vi "36DUT Plot From Spread Sheet Ver1.5a.vi"(6 "Plot":T1(ring), 7 "No of Rows":i32=10496, 8 "error in (no error)":errorcluster, 10 "Bank":i32(ring) items=["C1", "C2", "C3", "D_C1", "D_C2", "D_C3", "D_B1_C1", "D_B1_C2", "D_B1_C3"], 11 "file path (dialog if empty)":path) -> (0 "error out":errorcluster, 3 "Delta C_Min Plot":dbl[][](graph) caption="(Y) Multi Plot 2")   [LabVIEW 2012]
uses:
  <vilib>/Utility/file.llb/Read From Spreadsheet File (string).vi
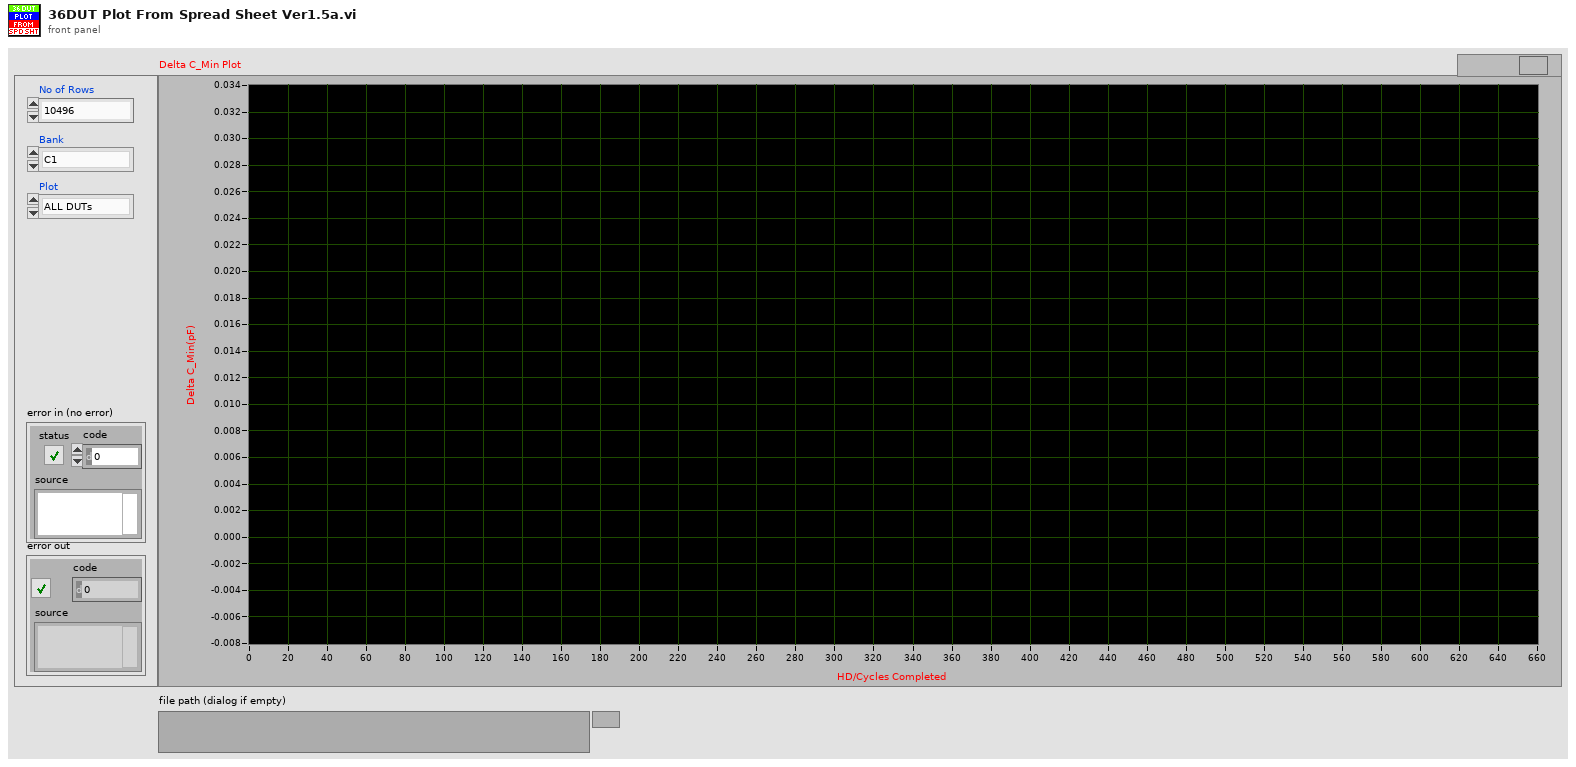
[diagram p1: front panel]
types:
  T1 = enum16{"ALL DUTs", "DUT 01", "DUT 02", "DUT 03", "DUT 04", "DUT 05", "DUT 06", "DUT 07", "DUT 08", "DUT 09", "DUT 10", "DUT 11", "DUT 12", "DUT 13", "DUT 14", "DUT 15", "DUT 16", "DUT 17", "DUT 18", "DUT 19", "DUT 20", "DUT 21", "DUT 22", "DUT 23", "DUT 24", "DUT 25", "DUT 26", "DUT 27", "DUT 28", "DUT 29", "DUT 30", "DUT 31", "DUT 32", "DUT 33", "DUT 34", "DUT 35", "DUT 36"}
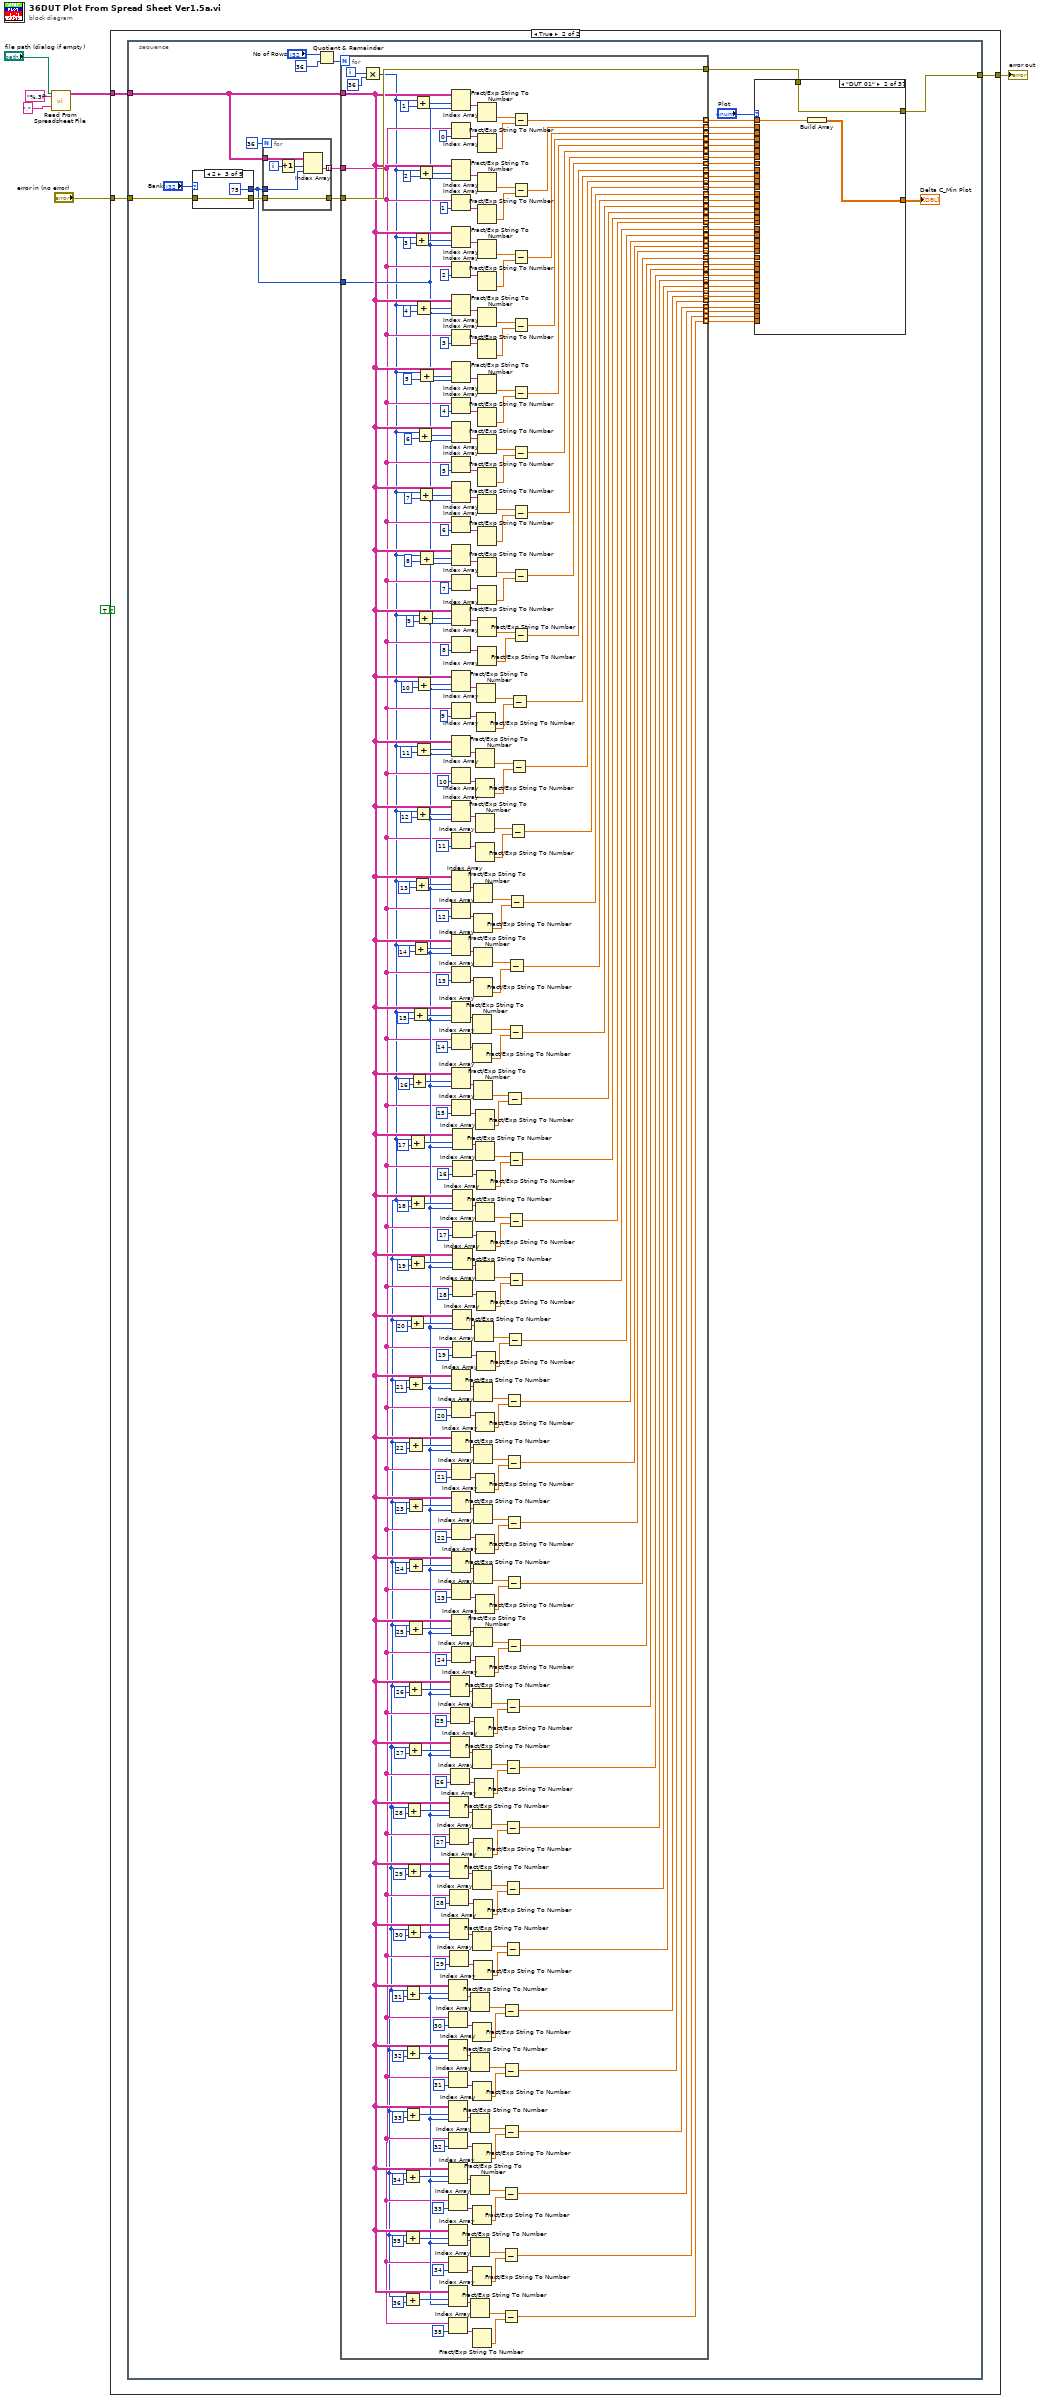
[diagram p0: block diagram]
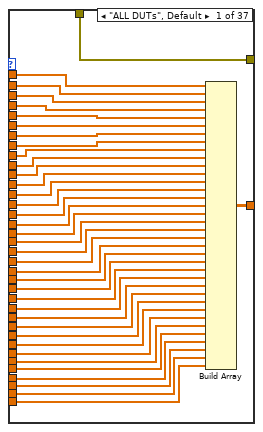
[diagram p3: hidden frame]
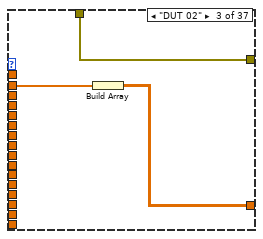
[diagram p4: hidden frame]
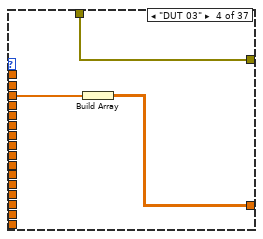
[diagram p5: hidden frame]
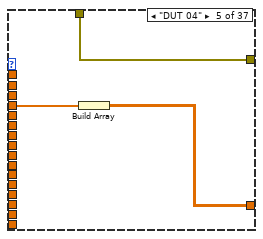
[diagram p6: hidden frame]
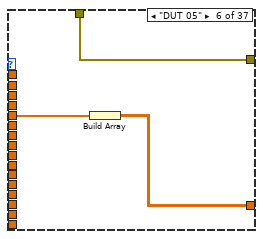
[diagram p7: hidden frame]
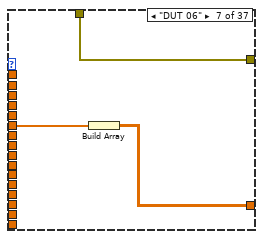
[diagram p8: hidden frame]
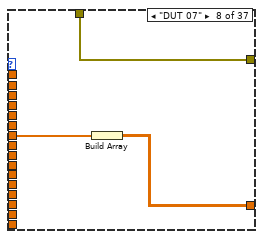
[diagram p9: hidden frame]
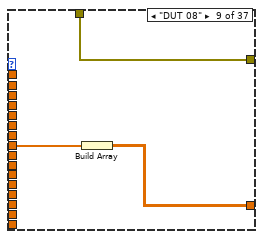
[diagram p10: hidden frame]
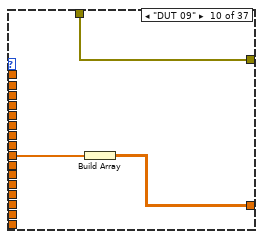
[diagram p11: hidden frame]
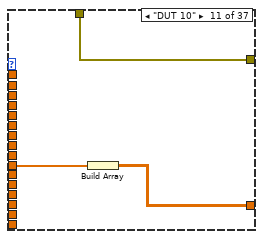
[diagram p12: hidden frame]
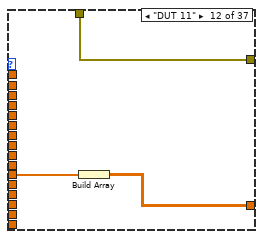
[diagram p13: hidden frame]
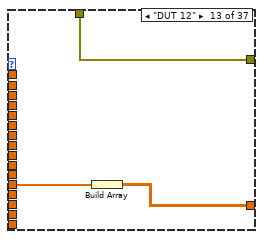
[diagram p14: hidden frame]
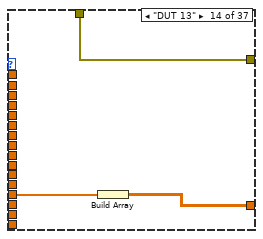
[diagram p15: hidden frame]
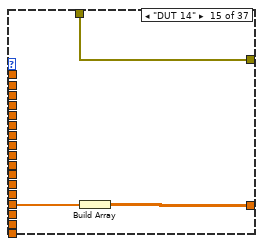
[diagram p16: hidden frame]
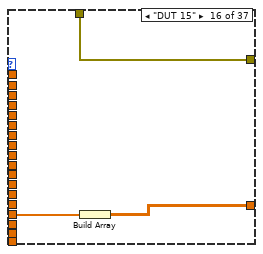
[diagram p17: hidden frame]
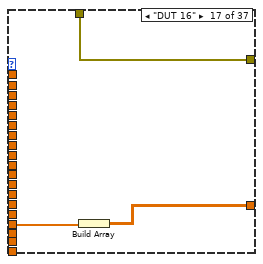
[diagram p18: hidden frame]
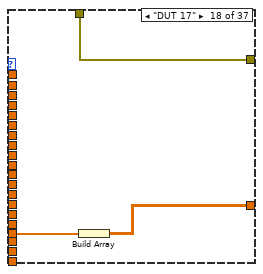
[diagram p19: hidden frame]
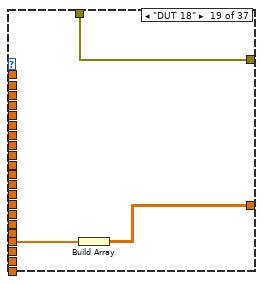
[diagram p20: hidden frame]
diagram:
  n1 = call-poly <vilib>:"Read From Spreadsheet File.vi"("delimiter (\\t)"="," ("delimiter (\\t)"), "format (%s)"="%.3f" ("format (%.3f)"), "file path (dialog if empty)"="file path (dialog if empty)") -> ("all rows"=w1:string[][])  [unwired: 4 in, 4 out]
  n2 = case shown="True" TRUE {
    tunnel: "error in (no error)" -> [w8 w11]
    tunnel: [w8 w10] -> w6
    tunnel: w1 -> [_ w9]
    frame False {
    }
    frame True {
      n3 = stacked-sequence {
        tunnel: w11 -> [w38]
        tunnel: [w33] -> w10
        tunnel: w9 -> [w12]
        frame #0 {
          n4 = case shown="2" "Bank" {
            tunnel: [5 40 75 119 120 121 35 36 37] -> w34
            tunnel: [w209 w211 w213 w216 w218 w220 w221 w223 w225] -> w35
            tunnel: w38 -> [w209 w211 w213 w216 w218 w220 w221 w223 w225]
            frame 0, Default {
            }
            frame 1 {
            }
            frame 2 {
            }
            frame 3 {
            }
            frame 4 {
            }
            frame 5 {
            }
            frame 6 {
            }
            frame 7 {
            }
            frame 8 {
            }
          }
          n5 = for {
            N: 36 -> [_]
            tunnel: w12 -> [w527]
            tunnel: [w526] -> w61 mode=indexing
            tunnel: w34 -> [w522]
            tunnel: [w523] -> w37
            tunnel: w35 -> [w523]
            i -> [w525]
            n6 = Increment(x=w525) -> (x+1=w524:i32)
            n7 = Index Array(array=w527, index (row)=w524, index (col)=w522) -> (element=w526:string)
          }
          n8 = Quotient & Remainder(x="No of Rows", y=36) -> (floor(x/y)=w57:i32)  [unwired: 1 out]
          n9 = for {
            N: w57 -> [_]
            tunnel: w12 -> [w250]
            tunnel: w61 -> [w248]
            tunnel: [w408] -> w55 mode=indexing
            tunnel: [w407] -> w54 mode=indexing
            tunnel: [w406] -> w53 mode=indexing
            tunnel: [w405] -> w52 mode=indexing
            tunnel: [w404] -> w51 mode=indexing
            tunnel: [w403] -> w50 mode=indexing
            tunnel: [w402] -> w49 mode=indexing
            tunnel: [w401] -> w48 mode=indexing
            tunnel: [w400] -> w47 mode=indexing
            tunnel: [w399] -> w46 mode=indexing
            tunnel: [w398] -> w45 mode=indexing
            tunnel: [w397] -> w44 mode=indexing
            tunnel: [w396] -> w43 mode=indexing
            tunnel: [w395] -> w42 mode=indexing
            tunnel: [w394] -> w41 mode=indexing
            tunnel: [w393] -> w40 mode=indexing
            tunnel: w37 -> [w392]
            tunnel: [w392] -> w36
            tunnel: w34 -> [w249]
            tunnel: [w247] -> w32 mode=indexing
            tunnel: [w246] -> w31 mode=indexing
            tunnel: [w245] -> w30 mode=indexing
            tunnel: [w244] -> w29 mode=indexing
            tunnel: [w243] -> w28 mode=indexing
            tunnel: [w242] -> w27 mode=indexing
            tunnel: [w241] -> w26 mode=indexing
            tunnel: [w240] -> w25 mode=indexing
            tunnel: [w239] -> w24 mode=indexing
            tunnel: [w238] -> w23 mode=indexing
            tunnel: [w237] -> w22 mode=indexing
            tunnel: [w236] -> w21 mode=indexing
            tunnel: [w235] -> w20 mode=indexing
            tunnel: [w234] -> w19 mode=indexing
            tunnel: [w233] -> w18 mode=indexing
            tunnel: [w232] -> w17 mode=indexing
            tunnel: [w231] -> w16 mode=indexing
            tunnel: [w230] -> w15 mode=indexing
            tunnel: [w229] -> w14 mode=indexing
            tunnel: [w228] -> w13 mode=indexing
            i -> [w391]
            n10 = Multiply(x=w391, y=36) -> (x*y=w227:i32)
            n11 = Add(x=w227, y=34) -> (x+y=w271:i32)
            n12 = Add(x=w227, y=35) -> (x+y=w258:i32)
            n13 = Add(x=w227, y=36) -> (x+y=w257:i32)
            n14 = Add(x=w227, y=31) -> (x+y=w286:i32)
            n15 = Add(x=w227, y=32) -> (x+y=w285:i32)
            n16 = Add(x=w227, y=33) -> (x+y=w272:i32)
            n17 = Add(x=w227, y=28) -> (x+y=w313:i32)
            n18 = Add(x=w227, y=29) -> (x+y=w300:i32)
            n19 = Add(x=w227, y=30) -> (x+y=w299:i32)
            n20 = Add(x=w227, y=26) -> (x+y=w327:i32)
            n21 = Add(x=w227, y=27) -> (x+y=w314:i32)
            n22 = Add(x=w227, y=21) -> (x+y=w356:i32)
            n23 = Add(x=w227, y=22) -> (x+y=w355:i32)
            n24 = Add(x=w227, y=23) -> (x+y=w342:i32)
            n25 = Add(x=w227, y=24) -> (x+y=w341:i32)
            n26 = Add(x=w227, y=25) -> (x+y=w328:i32)
            n27 = Add(x=w227, y=20) -> (x+y=w369:i32)
            n28 = Add(x=w227, y=17) -> (x+y=w384:i32)
            n29 = Add(x=w227, y=18) -> (x+y=w383:i32)
            n30 = Add(x=w227, y=19) -> (x+y=w370:i32)
            n31 = Add(x=w227, y=16) -> (x+y=w413:i32)
            n32 = Add(x=w227, y=15) -> (x+y=w418:i32)
            n33 = Add(x=w227, y=14) -> (x+y=w427:i32)
            n34 = Add(x=w227, y=13) -> (x+y=w432:i32)
            n35 = Add(x=w227, y=3) -> (x+y=w487:i32)
            n36 = Add(x=w227, y=1) -> (x+y=w509:i32)
            n37 = Add(x=w227, y=12) -> (x+y=w441:i32)
            n38 = Add(x=w227, y=4) -> (x+y=w486:i32)
            n39 = Add(x=w227, y=11) -> (x+y=w446:i32)
            n40 = Add(x=w227, y=10) -> (x+y=w455:i32)
            n41 = Add(x=w227, y=6) -> (x+y=w472:i32)
            n42 = Add(x=w227, y=9) -> (x+y=w502:i32)
            n43 = Add(x=w227, y=2) -> (x+y=w506:i32)
            n44 = Add(x=w227, y=7) -> (x+y=w465:i32)
            n45 = Add(x=w227, y=5) -> (x+y=w479:i32)
            n46 = Add(x=w227, y=8) -> (x+y=w459:i32)
            n47 = Index Array(array=w250, index (row)=w271, index (col)=w249) -> (element=w266:string)
            n48 = Index Array(array=w248, index=33) -> (element=w268:string)
            n49 = Index Array(array=w250, index (row)=w258, index (col)=w249) -> (element=w263:string)
            n50 = Index Array(array=w248, index=34) -> (element=w261:string)
            n51 = Index Array(array=w250, index (row)=w257, index (col)=w249) -> (element=w252:string)
            n52 = Index Array(array=w248, index=35) -> (element=w254:string)
            n53 = Index Array(array=w250, index (row)=w286, index (col)=w249) -> (element=w291:string)
            n54 = Index Array(array=w248, index=30) -> (element=w289:string)
            n55 = Index Array(array=w250, index (row)=w285, index (col)=w249) -> (element=w280:string)
            n56 = Index Array(array=w248, index=31) -> (element=w282:string)
            n57 = Index Array(array=w250, index (row)=w272, index (col)=w249) -> (element=w277:string)
            n58 = Index Array(array=w248, index=32) -> (element=w275:string)
            n59 = Index Array(array=w250, index (row)=w313, index (col)=w249) -> (element=w308:string)
            n60 = Index Array(array=w248, index=27) -> (element=w310:string)
            n61 = Index Array(array=w250, index (row)=w300, index (col)=w249) -> (element=w305:string)
            n62 = Index Array(array=w248, index=28) -> (element=w303:string)
            n63 = Index Array(array=w250, index (row)=w299, index (col)=w249) -> (element=w294:string)
            n64 = Index Array(array=w248, index=29) -> (element=w296:string)
            n65 = Index Array(array=w250, index (row)=w327, index (col)=w249) -> (element=w322:string)
            n66 = Index Array(array=w248, index=25) -> (element=w324:string)
            n67 = Index Array(array=w250, index (row)=w314, index (col)=w249) -> (element=w319:string)
            n68 = Index Array(array=w248, index=26) -> (element=w317:string)
            n69 = Index Array(array=w250, index (row)=w356, index (col)=w249) -> (element=w361:string)
            n70 = Index Array(array=w248, index=20) -> (element=w359:string)
            n71 = Index Array(array=w250, index (row)=w355, index (col)=w249) -> (element=w350:string)
            n72 = Index Array(array=w248, index=21) -> (element=w352:string)
            n73 = Index Array(array=w250, index (row)=w342, index (col)=w249) -> (element=w347:string)
            n74 = Index Array(array=w248, index=22) -> (element=w345:string)
            n75 = Index Array(array=w250, index (row)=w341, index (col)=w249) -> (element=w336:string)
            n76 = Index Array(array=w248, index=23) -> (element=w338:string)
            n77 = Index Array(array=w250, index (row)=w328, index (col)=w249) -> (element=w333:string)
            n78 = Index Array(array=w248, index=24) -> (element=w331:string)
            n79 = Index Array(array=w250, index (row)=w509, index (col)=w249) -> (element=w520:string)
            n80 = Index Array(array=w248, index=0) -> (element=w518:string)
            n81 = Index Array(array=w250, index (row)=w506, index (col)=w249) -> (element=w511:string)
            n82 = Index Array(array=w248, index=1) -> (element=w513:string)
            n83 = Index Array(array=w250, index (row)=w487, index (col)=w249) -> (element=w499:string)
            n84 = Index Array(array=w248, index=2) -> (element=w497:string)
            n85 = Index Array(array=w250, index (row)=w486, index (col)=w249) -> (element=w489:string)
            n86 = Index Array(array=w248, index=3) -> (element=w491:string)
            n87 = Index Array(array=w250, index (row)=w479, index (col)=w249) -> (element=w485:string)
            n88 = Index Array(array=w248, index=4) -> (element=w483:string)
            n89 = Index Array(array=w250, index (row)=w472, index (col)=w249) -> (element=w474:string)
            n90 = Index Array(array=w248, index=5) -> (element=w476:string)
            n91 = Index Array(array=w250, index (row)=w465, index (col)=w249) -> (element=w471:string)
            n92 = Index Array(array=w248, index=6) -> (element=w469:string)
            n93 = Index Array(array=w250, index (row)=w459, index (col)=w249) -> (element=w458:string)
            n94 = Index Array(array=w248, index=7) -> (element=w462:string)
            n95 = Index Array(array=w250, index (row)=w502, index (col)=w249) -> (element=w505:string)
            n96 = Index Array(array=w248, index=8) -> (element=w503:string)
            n97 = Index Array(array=w250, index (row)=w455, index (col)=w249) -> (element=w452:string)
            n98 = Index Array(array=w248, index=9) -> (element=w454:string)
            n99 = Index Array(array=w250, index (row)=w446, index (col)=w249) -> (element=w449:string)
            n100 = Index Array(array=w248, index=10) -> (element=w447:string)
            n101 = Index Array(array=w250, index (row)=w441, index (col)=w249) -> (element=w438:string)
            n102 = Index Array(array=w248, index=11) -> (element=w440:string)
            n103 = Index Array(array=w250, index (row)=w432, index (col)=w249) -> (element=w435:string)
            n104 = Index Array(array=w248, index=12) -> (element=w433:string)
            n105 = Index Array(array=w250, index (row)=w427, index (col)=w249) -> (element=w424:string)
            n106 = Index Array(array=w248, index=13) -> (element=w426:string)
            n107 = Index Array(array=w250, index (row)=w418, index (col)=w249) -> (element=w421:string)
            n108 = Index Array(array=w248, index=14) -> (element=w419:string)
            n109 = Index Array(array=w250, index (row)=w413, index (col)=w249) -> (element=w410:string)
            n110 = Index Array(array=w248, index=15) -> (element=w412:string)
            n111 = Index Array(array=w250, index (row)=w369, index (col)=w249) -> (element=w364:string)
            n112 = Index Array(array=w248, index=19) -> (element=w366:string)
            n113 = Index Array(array=w250, index (row)=w384, index (col)=w249) -> (element=w389:string)
            n114 = Index Array(array=w248, index=16) -> (element=w387:string)
            n115 = Index Array(array=w250, index (row)=w383, index (col)=w249) -> (element=w378:string)
            n116 = Index Array(array=w248, index=17) -> (element=w380:string)
            n117 = Index Array(array=w250, index (row)=w370, index (col)=w249) -> (element=w375:string)
            n118 = Index Array(array=w248, index=18) -> (element=w373:string)
            n119 = Fract/Exp String To Number(string=w266) -> (number=w269:dbl)  [unwired: 3 in, 1 out]
            n120 = Fract/Exp String To Number(string=w263) -> (number=w260:dbl)  [unwired: 3 in, 1 out]
            n121 = Fract/Exp String To Number(string=w252) -> (number=w255:dbl)  [unwired: 3 in, 1 out]
            n122 = Fract/Exp String To Number(string=w291) -> (number=w288:dbl)  [unwired: 3 in, 1 out]
            n123 = Fract/Exp String To Number(string=w280) -> (number=w283:dbl)  [unwired: 3 in, 1 out]
            n124 = Fract/Exp String To Number(string=w277) -> (number=w274:dbl)  [unwired: 3 in, 1 out]
            n125 = Fract/Exp String To Number(string=w308) -> (number=w311:dbl)  [unwired: 3 in, 1 out]
            n126 = Fract/Exp String To Number(string=w305) -> (number=w302:dbl)  [unwired: 3 in, 1 out]
            n127 = Fract/Exp String To Number(string=w294) -> (number=w297:dbl)  [unwired: 3 in, 1 out]
            n128 = Fract/Exp String To Number(string=w268) -> (number=w270:dbl)  [unwired: 3 in, 1 out]
            n129 = Fract/Exp String To Number(string=w261) -> (number=w259:dbl)  [unwired: 3 in, 1 out]
            n130 = Fract/Exp String To Number(string=w254) -> (number=w256:dbl)  [unwired: 3 in, 1 out]
            n131 = Fract/Exp String To Number(string=w421) -> (number=w417:dbl)  [unwired: 3 in, 1 out]
            n132 = Fract/Exp String To Number(string=w419) -> (number=w416:dbl)  [unwired: 3 in, 1 out]
            n133 = Fract/Exp String To Number(string=w322) -> (number=w325:dbl)  [unwired: 3 in, 1 out]
            n134 = Fract/Exp String To Number(string=w319) -> (number=w316:dbl)  [unwired: 3 in, 1 out]
            n135 = Fract/Exp String To Number(string=w289) -> (number=w287:dbl)  [unwired: 3 in, 1 out]
            n136 = Fract/Exp String To Number(string=w282) -> (number=w284:dbl)  [unwired: 3 in, 1 out]
            n137 = Fract/Exp String To Number(string=w275) -> (number=w273:dbl)  [unwired: 3 in, 1 out]
            n138 = Fract/Exp String To Number(string=w424) -> (number=w428:dbl)  [unwired: 3 in, 1 out]
            n139 = Fract/Exp String To Number(string=w426) -> (number=w429:dbl)  [unwired: 3 in, 1 out]
            n140 = Fract/Exp String To Number(string=w361) -> (number=w358:dbl)  [unwired: 3 in, 1 out]
            n141 = Fract/Exp String To Number(string=w350) -> (number=w353:dbl)  [unwired: 3 in, 1 out]
            n142 = Fract/Exp String To Number(string=w347) -> (number=w344:dbl)  [unwired: 3 in, 1 out]
            n143 = Fract/Exp String To Number(string=w336) -> (number=w339:dbl)  [unwired: 3 in, 1 out]
            n144 = Fract/Exp String To Number(string=w333) -> (number=w330:dbl)  [unwired: 3 in, 1 out]
            n145 = Fract/Exp String To Number(string=w435) -> (number=w431:dbl)  [unwired: 3 in, 1 out]
            n146 = Fract/Exp String To Number(string=w433) -> (number=w430:dbl)  [unwired: 3 in, 1 out]
            n147 = Fract/Exp String To Number(string=w410) -> (number=w414:dbl)  [unwired: 3 in, 1 out]
            n148 = Fract/Exp String To Number(string=w310) -> (number=w312:dbl)  [unwired: 3 in, 1 out]
            n149 = Fract/Exp String To Number(string=w303) -> (number=w301:dbl)  [unwired: 3 in, 1 out]
            n150 = Fract/Exp String To Number(string=w296) -> (number=w298:dbl)  [unwired: 3 in, 1 out]
            n151 = Fract/Exp String To Number(string=w364) -> (number=w367:dbl)  [unwired: 3 in, 1 out]
            n152 = Fract/Exp String To Number(string=w324) -> (number=w326:dbl)  [unwired: 3 in, 1 out]
            n153 = Fract/Exp String To Number(string=w317) -> (number=w315:dbl)  [unwired: 3 in, 1 out]
            n154 = Fract/Exp String To Number(string=w438) -> (number=w442:dbl)  [unwired: 3 in, 1 out]
            n155 = Fract/Exp String To Number(string=w440) -> (number=w443:dbl)  [unwired: 3 in, 1 out]
            n156 = Fract/Exp String To Number(string=w389) -> (number=w386:dbl)  [unwired: 3 in, 1 out]
            n157 = Fract/Exp String To Number(string=w378) -> (number=w381:dbl)  [unwired: 3 in, 1 out]
            n158 = Fract/Exp String To Number(string=w375) -> (number=w372:dbl)  [unwired: 3 in, 1 out]
            n159 = Fract/Exp String To Number(string=w359) -> (number=w357:dbl)  [unwired: 3 in, 1 out]
            n160 = Fract/Exp String To Number(string=w352) -> (number=w354:dbl)  [unwired: 3 in, 1 out]
            n161 = Fract/Exp String To Number(string=w345) -> (number=w343:dbl)  [unwired: 3 in, 1 out]
            n162 = Fract/Exp String To Number(string=w338) -> (number=w340:dbl)  [unwired: 3 in, 1 out]
            n163 = Fract/Exp String To Number(string=w331) -> (number=w329:dbl)  [unwired: 3 in, 1 out]
            n164 = Fract/Exp String To Number(string=w449) -> (number=w445:dbl)  [unwired: 3 in, 1 out]
            n165 = Fract/Exp String To Number(string=w447) -> (number=w444:dbl)  [unwired: 3 in, 1 out]
            n166 = Fract/Exp String To Number(string=w412) -> (number=w415:dbl)  [unwired: 3 in, 1 out]
            n167 = Fract/Exp String To Number(string=w452) -> (number=w456:dbl)  [unwired: 3 in, 1 out]
            n168 = Fract/Exp String To Number(string=w454) -> (number=w457:dbl)  [unwired: 3 in, 1 out]
            n169 = Fract/Exp String To Number(string=w366) -> (number=w368:dbl)  [unwired: 3 in, 1 out]
            n170 = Fract/Exp String To Number(string=w387) -> (number=w385:dbl)  [unwired: 3 in, 1 out]
            n171 = Fract/Exp String To Number(string=w380) -> (number=w382:dbl)  [unwired: 3 in, 1 out]
            n172 = Fract/Exp String To Number(string=w373) -> (number=w371:dbl)  [unwired: 3 in, 1 out]
            n173 = Fract/Exp String To Number(string=w520) -> (number=w517:dbl)  [unwired: 3 in, 1 out]
            n174 = Fract/Exp String To Number(string=w518) -> (number=w516:dbl)  [unwired: 3 in, 1 out]
            n175 = Fract/Exp String To Number(string=w511) -> (number=w514:dbl)  [unwired: 3 in, 1 out]
            n176 = Fract/Exp String To Number(string=w513) -> (number=w515:dbl)  [unwired: 3 in, 1 out]
            n177 = Fract/Exp String To Number(string=w499) -> (number=w496:dbl)  [unwired: 3 in, 1 out]
            n178 = Fract/Exp String To Number(string=w497) -> (number=w495:dbl)  [unwired: 3 in, 1 out]
            n179 = Fract/Exp String To Number(string=w489) -> (number=w492:dbl)  [unwired: 3 in, 1 out]
            n180 = Fract/Exp String To Number(string=w491) -> (number=w493:dbl)  [unwired: 3 in, 1 out]
            n181 = Fract/Exp String To Number(string=w485) -> (number=w482:dbl)  [unwired: 3 in, 1 out]
            n182 = Fract/Exp String To Number(string=w483) -> (number=w481:dbl)  [unwired: 3 in, 1 out]
            n183 = Fract/Exp String To Number(string=w474) -> (number=w477:dbl)  [unwired: 3 in, 1 out]
            n184 = Fract/Exp String To Number(string=w476) -> (number=w478:dbl)  [unwired: 3 in, 1 out]
            n185 = Fract/Exp String To Number(string=w471) -> (number=w468:dbl)  [unwired: 3 in, 1 out]
            n186 = Fract/Exp String To Number(string=w469) -> (number=w467:dbl)  [unwired: 3 in, 1 out]
            n187 = Fract/Exp String To Number(string=w458) -> (number=w463:dbl)  [unwired: 3 in, 1 out]
            n188 = Fract/Exp String To Number(string=w462) -> (number=w464:dbl)  [unwired: 3 in, 1 out]
            n189 = Fract/Exp String To Number(string=w505) -> (number=w501:dbl)  [unwired: 3 in, 1 out]
            n190 = Fract/Exp String To Number(string=w503) -> (number=w500:dbl)  [unwired: 3 in, 1 out]
            n191 = Subtract(x=w269, y=w270) -> (x-y=w230:dbl)
            n192 = Subtract(x=w260, y=w259) -> (x-y=w229:dbl)
            n193 = Subtract(x=w255, y=w256) -> (x-y=w228:dbl)
            n194 = Subtract(x=w288, y=w287) -> (x-y=w233:dbl)
            n195 = Subtract(x=w283, y=w284) -> (x-y=w232:dbl)
            n196 = Subtract(x=w274, y=w273) -> (x-y=w231:dbl)
            n197 = Subtract(x=w311, y=w312) -> (x-y=w236:dbl)
            n198 = Subtract(x=w302, y=w301) -> (x-y=w235:dbl)
            n199 = Subtract(x=w297, y=w298) -> (x-y=w234:dbl)
            n200 = Subtract(x=w325, y=w326) -> (x-y=w238:dbl)
            n201 = Subtract(x=w316, y=w315) -> (x-y=w237:dbl)
            n202 = Subtract(x=w358, y=w357) -> (x-y=w243:dbl)
            n203 = Subtract(x=w353, y=w354) -> (x-y=w242:dbl)
            n204 = Subtract(x=w344, y=w343) -> (x-y=w241:dbl)
            n205 = Subtract(x=w339, y=w340) -> (x-y=w240:dbl)
            n206 = Subtract(x=w330, y=w329) -> (x-y=w239:dbl)
            n207 = Subtract(x=w414, y=w415) -> (x-y=w393:dbl)
            n208 = Subtract(x=w367, y=w368) -> (x-y=w244:dbl)
            n209 = Subtract(x=w417, y=w416) -> (x-y=w394:dbl)
            n210 = Subtract(x=w386, y=w385) -> (x-y=w247:dbl)
            n211 = Subtract(x=w381, y=w382) -> (x-y=w246:dbl)
            n212 = Subtract(x=w372, y=w371) -> (x-y=w245:dbl)
            n213 = Subtract(x=w428, y=w429) -> (x-y=w395:dbl)
            n214 = Subtract(x=w431, y=w430) -> (x-y=w396:dbl)
            n215 = Subtract(x=w442, y=w443) -> (x-y=w397:dbl)
            n216 = Subtract(x=w445, y=w444) -> (x-y=w398:dbl)
            n217 = Subtract(x=w456, y=w457) -> (x-y=w399:dbl)
            n218 = Subtract(x=w517, y=w516) -> (x-y=w408:dbl)
            n219 = Subtract(x=w514, y=w515) -> (x-y=w407:dbl)
            n220 = Subtract(x=w496, y=w495) -> (x-y=w406:dbl)
            n221 = Subtract(x=w492, y=w493) -> (x-y=w405:dbl)
            n222 = Subtract(x=w482, y=w481) -> (x-y=w404:dbl)
            n223 = Subtract(x=w477, y=w478) -> (x-y=w403:dbl)
            n224 = Subtract(x=w468, y=w467) -> (x-y=w402:dbl)
            n225 = Subtract(x=w463, y=w464) -> (x-y=w401:dbl)
            n226 = Subtract(x=w501, y=w500) -> (x-y=w400:dbl)
          }
          n227 = case shown="\"DUT 01\"" "Plot" {
            tunnel: w55 -> [w100 w103 _ _ _ _ _ _ _ _ _ _ _ _ _ _ _ _ _ _ _ _ _ _ _ _ _ _ _ _ _ _ _ _ _ _ _]
            tunnel: w54 -> [w99 _ w105 _ _ _ _ _ _ _ _ _ _ _ _ _ _ _ _ _ _ _ _ _ _ _ _ _ _ _ _ _ _ _ _ _ _]
            tunnel: w53 -> [w98 _ _ w109 _ _ _ _ _ _ _ _ _ _ _ _ _ _ _ _ _ _ _ _ _ _ _ _ _ _ _ _ _ _ _ _ _]
            tunnel: w52 -> [w97 _ _ _ w111 _ _ _ _ _ _ _ _ _ _ _ _ _ _ _ _ _ _ _ _ _ _ _ _ _ _ _ _ _ _ _ _]
            tunnel: w51 -> [w96 _ _ _ _ w115 _ _ _ _ _ _ _ _ _ _ _ _ _ _ _ _ _ _ _ _ _ _ _ _ _ _ _ _ _ _ _]
            tunnel: w50 -> [w95 _ _ _ _ _ w117 _ _ _ _ _ _ _ _ _ _ _ _ _ _ _ _ _ _ _ _ _ _ _ _ _ _ _ _ _ _]
            tunnel: w49 -> [w94 _ _ _ _ _ _ w120 _ _ _ _ _ _ _ _ _ _ _ _ _ _ _ _ _ _ _ _ _ _ _ _ _ _ _ _ _]
            tunnel: w48 -> [w93 _ _ _ _ _ _ _ w124 _ _ _ _ _ _ _ _ _ _ _ _ _ _ _ _ _ _ _ _ _ _ _ _ _ _ _ _]
            tunnel: w47 -> [w92 _ _ _ _ _ _ _ _ w127 _ _ _ _ _ _ _ _ _ _ _ _ _ _ _ _ _ _ _ _ _ _ _ _ _ _ _]
            tunnel: w46 -> [w91 _ _ _ _ _ _ _ _ _ w130 _ _ _ _ _ _ _ _ _ _ _ _ _ _ _ _ _ _ _ _ _ _ _ _ _ _]
            tunnel: w45 -> [w90 _ _ _ _ _ _ _ _ _ _ w133 _ _ _ _ _ _ _ _ _ _ _ _ _ _ _ _ _ _ _ _ _ _ _ _ _]
            tunnel: w44 -> [w89 _ _ _ _ _ _ _ _ _ _ _ w136 _ _ _ _ _ _ _ _ _ _ _ _ _ _ _ _ _ _ _ _ _ _ _ _]
            tunnel: w43 -> [w88 _ _ _ _ _ _ _ _ _ _ _ _ w139 _ _ _ _ _ _ _ _ _ _ _ _ _ _ _ _ _ _ _ _ _ _ _]
            tunnel: w42 -> [w87 _ _ _ _ _ _ _ _ _ _ _ _ _ w142 _ _ _ _ _ _ _ _ _ _ _ _ _ _ _ _ _ _ _ _ _ _]
            tunnel: w41 -> [w86 _ _ _ _ _ _ _ _ _ _ _ _ _ _ w145 _ _ _ _ _ _ _ _ _ _ _ _ _ _ _ _ _ _ _ _ _]
            tunnel: w40 -> [w85 _ _ _ _ _ _ _ _ _ _ _ _ _ _ _ w147 _ _ _ _ _ _ _ _ _ _ _ _ _ _ _ _ _ _ _ _]
            tunnel: [w84 w102 w106 w108 w112 w114 w118 w121 w123 w126 w129 w132 w135 w138 w141 w144 w148 w151 w154 w157 w160 w163 w166 w169 w172 w175 w178 w181 w184 w187 w190 w193 w196 w199 w202 w205 w208] -> w39
            tunnel: w36 -> [w83 w101 w104 w107 w110 w113 w116 w119 w122 w125 w128 w131 w134 w137 w140 w143 w146 w150 w153 w156 w159 w162 w165 w168 w171 w174 w177 w180 w183 w186 w189 w192 w195 w198 w201 w204 w207]
            tunnel: [w83 w101 w104 w107 w110 w113 w116 w119 w122 w125 w128 w131 w134 w137 w140 w143 w146 w150 w153 w156 w159 w162 w165 w168 w171 w174 w177 w180 w183 w186 w189 w192 w195 w198 w201 w204 w207] -> w33
            tunnel: w32 -> [w82 _ _ _ _ _ _ _ _ _ _ _ _ _ _ _ _ w149 _ _ _ _ _ _ _ _ _ _ _ _ _ _ _ _ _ _ _]
            tunnel: w31 -> [w81 _ _ _ _ _ _ _ _ _ _ _ _ _ _ _ _ _ w152 _ _ _ _ _ _ _ _ _ _ _ _ _ _ _ _ _ _]
            tunnel: w30 -> [w80 _ _ _ _ _ _ _ _ _ _ _ _ _ _ _ _ _ _ w155 _ _ _ _ _ _ _ _ _ _ _ _ _ _ _ _ _]
            tunnel: w29 -> [w79 _ _ _ _ _ _ _ _ _ _ _ _ _ _ _ _ _ _ _ w158 _ _ _ _ _ _ _ _ _ _ _ _ _ _ _ _]
            tunnel: w28 -> [w78 _ _ _ _ _ _ _ _ _ _ _ _ _ _ _ _ _ _ _ _ w161 _ _ _ _ _ _ _ _ _ _ _ _ _ _ _]
            tunnel: w27 -> [w77 _ _ _ _ _ _ _ _ _ _ _ _ _ _ _ _ _ _ _ _ _ w164 _ _ _ _ _ _ _ _ _ _ _ _ _ _]
            tunnel: w26 -> [w76 _ _ _ _ _ _ _ _ _ _ _ _ _ _ _ _ _ _ _ _ _ _ w167 _ _ _ _ _ _ _ _ _ _ _ _ _]
            tunnel: w25 -> [w75 _ _ _ _ _ _ _ _ _ _ _ _ _ _ _ _ _ _ _ _ _ _ _ w170 _ _ _ _ _ _ _ _ _ _ _ _]
            tunnel: w24 -> [w74 _ _ _ _ _ _ _ _ _ _ _ _ _ _ _ _ _ _ _ _ _ _ _ _ w173 _ _ _ _ _ _ _ _ _ _ _]
            tunnel: w23 -> [w73 _ _ _ _ _ _ _ _ _ _ _ _ _ _ _ _ _ _ _ _ _ _ _ _ _ w176 _ _ _ _ _ _ _ _ _ _]
            tunnel: w22 -> [w72 _ _ _ _ _ _ _ _ _ _ _ _ _ _ _ _ _ _ _ _ _ _ _ _ _ _ w179 _ _ _ _ _ _ _ _ _]
            tunnel: w21 -> [w71 _ _ _ _ _ _ _ _ _ _ _ _ _ _ _ _ _ _ _ _ _ _ _ _ _ _ _ w182 _ _ _ _ _ _ _ _]
            tunnel: w20 -> [w70 _ _ _ _ _ _ _ _ _ _ _ _ _ _ _ _ _ _ _ _ _ _ _ _ _ _ _ _ w185 _ _ _ _ _ _ _]
            tunnel: w19 -> [w69 _ _ _ _ _ _ _ _ _ _ _ _ _ _ _ _ _ _ _ _ _ _ _ _ _ _ _ _ _ w188 _ _ _ _ _ _]
            tunnel: w18 -> [w68 _ _ _ _ _ _ _ _ _ _ _ _ _ _ _ _ _ _ _ _ _ _ _ _ _ _ _ _ _ _ w191 _ _ _ _ _]
            tunnel: w17 -> [w67 _ _ _ _ _ _ _ _ _ _ _ _ _ _ _ _ _ _ _ _ _ _ _ _ _ _ _ _ _ _ _ w194 _ _ _ _]
            tunnel: w16 -> [w66 _ _ _ _ _ _ _ _ _ _ _ _ _ _ _ _ _ _ _ _ _ _ _ _ _ _ _ _ _ _ _ _ w197 _ _ _]
            tunnel: w15 -> [w65 _ _ _ _ _ _ _ _ _ _ _ _ _ _ _ _ _ _ _ _ _ _ _ _ _ _ _ _ _ _ _ _ _ w200 _ _]
            tunnel: w14 -> [w64 _ _ _ _ _ _ _ _ _ _ _ _ _ _ _ _ _ _ _ _ _ _ _ _ _ _ _ _ _ _ _ _ _ _ w203 _]
            tunnel: w13 -> [w63 _ _ _ _ _ _ _ _ _ _ _ _ _ _ _ _ _ _ _ _ _ _ _ _ _ _ _ _ _ _ _ _ _ _ _ w206]
            frame "ALL DUTs", Default {
              n228 = Build Array(w100, w99, w98, w97, w96, w95, w94, w93, w92, w91, w90, w89, w88, w87, w86, w85, w82, w81, w80, w79, w78, w77, w76, w75, w74, w73, w72, w71, w70, w69, w68, w67, w66, w65, w64, w63) -> (w84:dbl[][])
            }
            frame "DUT 01" {
              n229 = Build Array(w103) -> (w102:dbl[][])
            }
            frame "DUT 02" {
              n230 = Build Array(w105) -> (w106:dbl[][])
            }
            frame "DUT 03" {
              n231 = Build Array(w109) -> (w108:dbl[][])
            }
            frame "DUT 04" {
              n232 = Build Array(w111) -> (w112:dbl[][])
            }
            frame "DUT 05" {
              n233 = Build Array(w115) -> (w114:dbl[][])
            }
            frame "DUT 06" {
              n234 = Build Array(w117) -> (w118:dbl[][])
            }
            frame "DUT 07" {
              n235 = Build Array(w120) -> (w121:dbl[][])
            }
            frame "DUT 08" {
              n236 = Build Array(w124) -> (w123:dbl[][])
            }
            frame "DUT 09" {
              n237 = Build Array(w127) -> (w126:dbl[][])
            }
            frame "DUT 10" {
              n238 = Build Array(w130) -> (w129:dbl[][])
            }
            frame "DUT 11" {
              n239 = Build Array(w133) -> (w132:dbl[][])
            }
            frame "DUT 12" {
              n240 = Build Array(w136) -> (w135:dbl[][])
            }
            frame "DUT 13" {
              n241 = Build Array(w139) -> (w138:dbl[][])
            }
            frame "DUT 14" {
              n242 = Build Array(w142) -> (w141:dbl[][])
            }
            frame "DUT 15" {
              n243 = Build Array(w145) -> (w144:dbl[][])
            }
            frame "DUT 16" {
              n244 = Build Array(w147) -> (w148:dbl[][])
            }
            frame "DUT 17" {
              n245 = Build Array(w149) -> (w151:dbl[][])
            }
            frame "DUT 18" {
              n246 = Build Array(w152) -> (w154:dbl[][])
            }
            frame "DUT 19" {
              n247 = Build Array(w155) -> (w157:dbl[][])
            }
            frame "DUT 20" {
              n248 = Build Array(w158) -> (w160:dbl[][])
            }
            frame "DUT 21" {
              n249 = Build Array(w161) -> (w163:dbl[][])
            }
            frame "DUT 22" {
              n250 = Build Array(w164) -> (w166:dbl[][])
            }
            frame "DUT 23" {
              n251 = Build Array(w167) -> (w169:dbl[][])
            }
            frame "DUT 24" {
              n252 = Build Array(w170) -> (w172:dbl[][])
            }
            frame "DUT 25" {
              n253 = Build Array(w173) -> (w175:dbl[][])
            }
            frame "DUT 26" {
              n254 = Build Array(w176) -> (w178:dbl[][])
            }
            frame "DUT 27" {
              n255 = Build Array(w179) -> (w181:dbl[][])
            }
            frame "DUT 28" {
              n256 = Build Array(w182) -> (w184:dbl[][])
            }
            frame "DUT 29" {
              n257 = Build Array(w185) -> (w187:dbl[][])
            }
            frame "DUT 30" {
              n258 = Build Array(w188) -> (w190:dbl[][])
            }
            frame "DUT 31" {
              n259 = Build Array(w191) -> (w193:dbl[][])
            }
            frame "DUT 32" {
              n260 = Build Array(w194) -> (w196:dbl[][])
            }
            frame "DUT 33" {
              n261 = Build Array(w197) -> (w199:dbl[][])
            }
            frame "DUT 34" {
              n262 = Build Array(w200) -> (w202:dbl[][])
            }
            frame "DUT 35" {
              n263 = Build Array(w203) -> (w205:dbl[][])
            }
            frame "DUT 36" {
              n264 = Build Array(w206) -> (w208:dbl[][])
            }
          }
          "Delta C_Min Plot" <- w39
        }
      }
    }
  }
  "error out" <- w6
